vi "Obtain Hwnd.vi"(0 "Py Doc in":refnum<class "Py Doc.lvclass">, 11 "error in (no error)":errorcluster) -> (4 "Py Doc in":refnum<class "Py Doc.lvclass">, 15 "error out":errorcluster)   [LabVIEW 2016, in "Py Doc.lvclass"]
uses:
  Py Doc.lvclass
  D:/git/LabVIEW-MDI/source code/Document/Document.lvclass
  Document.lvclass/Document.ctl
  Document.lvclass
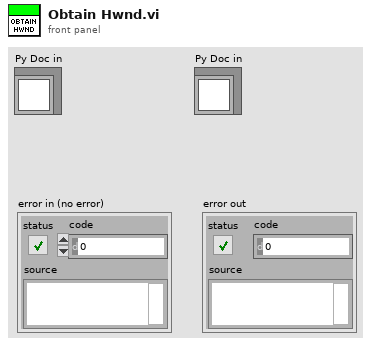
[diagram p1: front panel]
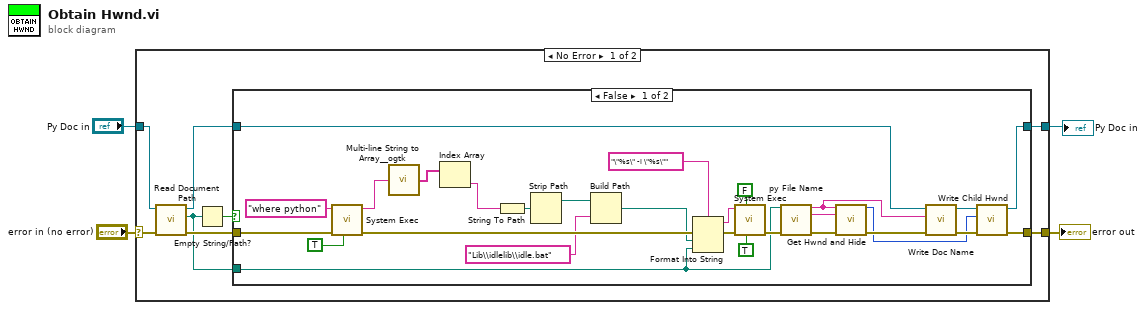
[diagram p0: block diagram]
diagram:
  n1 = case shown="No Error" "error in (no error)" {
    selector: "error in (no error)" -> [w10 w43]
    tunnel: "Py Doc in" -> [w8 w44]
    tunnel: [w12 w44] -> w1
    tunnel: [w11 w43] -> w3
    frame No Error {
      n2 = call "Read Document Path.vi"("error in (no error)"=w10, "Document in"=w8) -> ("error out"=w9:errorcluster, "Document Path"=w6:path, "Document out"=w7:refnum<class "Py Doc.lvclass">)  [unwired: 7 in]
      n3 = Empty String/Path?(string/path=w6) -> (empty?=w5:bool)
      n4 = case shown="False" w5 {
        tunnel: [w21 w41] -> w12
        tunnel: [w20 w42] -> w11
        tunnel: w9 -> [w19 w42]
        tunnel: w7 -> [w18 w41]
        tunnel: w6 -> [w17 _]
        frame False {
          n5 = call <vilib>:"System Exec.vi"("run minimized? (F)"=TRUE, "error in (no error)"=w19, "command line"="where python") -> ("error out"=w39:errorcluster, "standard output"=w15:string)  [unwired: 5 in, 2 out]
          n6 = call <userlib>:"Multi-line String to Array__ogtk.vi"("string"=w15) -> ("lines"=w16:string[])
          n7 = Index Array(array=w16) -> (element=w14:string)  [unwired: 1 in]
          n8 = String To Path(string=w14) -> (path=w35:path)
          n9 = Strip Path(path=w35) -> (stripped path=w36:path)  [unwired: 1 out]
          n10 = Build Path(base path=w36, name or relative path="Lib\\idlelib\\idle.bat") -> (appended path=w38:path)
          n11 = Format Into String(format string="\"%s\" -i \"%s\"", error in=w39, w38, w17) -> (resulting string=w23:string, error out=w22:errorcluster)  [unwired: 1 in]
          n12 = call <vilib>:"System Exec.vi"("run minimized? (F)"=TRUE, "wait until completion? (T)"=FALSE, "error in (no error)"=w22, "command line"=w23) -> ("error out"=w28:errorcluster)  [unwired: 4 in, 3 out]
          n13 = call "py File Name.vi"("Path"=w17, "error in (no error)"=w28) -> ("Doc Name"=w29:string, "Shell Name"=w40:string, "error out"=w26:errorcluster)  [unwired: 11 in]
          n14 = call "Get Hwnd and Hide.vi"("Doc Name"=w29, "Shell Name"=w40, "error in (no error)"=w26) -> ("hwnd"=w30:u32, "error out"=w33:errorcluster)  [unwired: 10 in, 1 out]
          n15 = call "Write Doc Name.vi"("error in (no error)"=w33, "Doc Name"=w29, "Document in"=w18) -> ("error out"=w32:errorcluster, "Document out"=w31:refnum<class "Py Doc.lvclass">)  [unwired: 7 in]
          n16 = call "Write Child Hwnd.vi"("error in (no error)"=w32, "Child Hwnd"=w30, "Document in"=w31) -> ("error out"=w20:errorcluster, "Document out"=w21:refnum<class "Py Doc.lvclass">)  [unwired: 7 in]
        }
        frame True {
        }
      }
    }
    frame Error {
    }
  }
  "error out" <- w3
  "Py Doc in" <- w1
